vi "Send Message (Single).vi"(8 "error in (no error)":errorcluster, 9 "Delay Seconds":i32, 10 "Message Body":string, 11 "SQS in":refnum<class "Queue.lvclass">) -> (0 "error out":errorcluster, 1 "Message Body MD5":string, 2 "Message ID":string, 3 "SQS out":refnum<class "Queue.lvclass">)   [LabVIEW 2015, in "NI_AWS_SQS.lvlib" / "Queue.lvclass"]
uses:
  Queue.lvclass
  Core/HTTP Request/Name Value Pair.ctl
  Core/HTTP Request/Request Options.ctl
  Queue.lvclass/Queue.ctl
  Read Account Number.vi
  Read Name.vi
  Core/HTTP Request/HTTP Request.lvclass
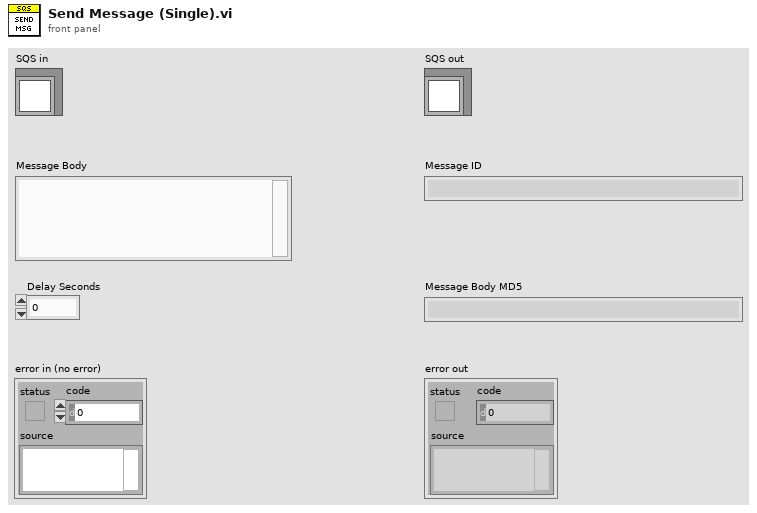
[diagram p1: front panel]
types:
  T1 = typedef "NI_AWS_Core.lvlib/HTTP Request.lvclass/Name Value Pair.ctl" = cluster{"name":string, "value":string}
  T2 = typedef "NI_AWS_Core.lvlib/HTTP Request.lvclass/Request Options.ctl" = cluster{"request headers":T1[], "request parameters":T1[], "request body":string}
  T3 = typedef "NI_AWS_Core.lvlib/HTTP Request.lvclass/Response.ctl" = cluster{"Headers":string, "Body":string}
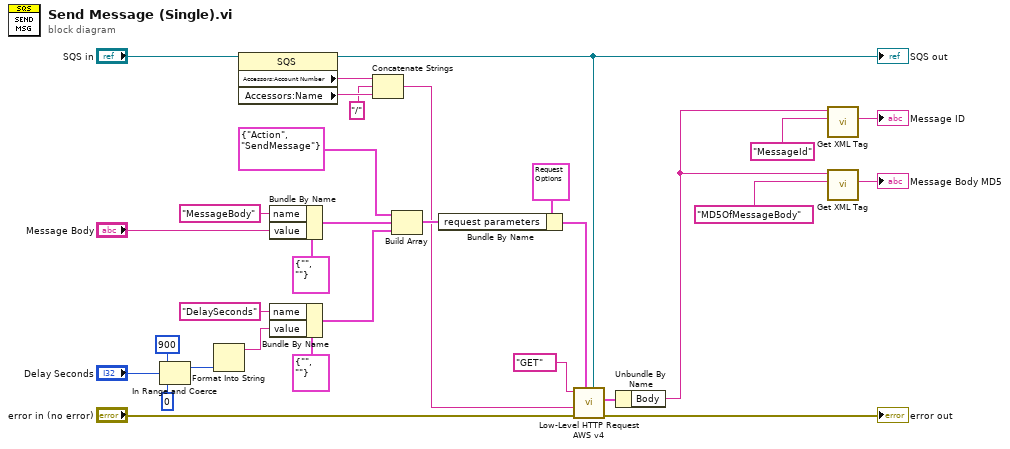
[diagram p0: block diagram]
diagram:
  n1 = In Range and Coerce(upper limit=900, x="Delay Seconds", lower limit=0) -> (coerced(x)=w3:i32)  [unwired: 1 out]
  n2 = Format Into String(w3) -> (resulting string=w5:string)  [unwired: 3 in, 1 out]
  n3 = property class="SQS"(reference="SQS in") -> (reference out=w22:refnum<class "Queue.lvclass">, "Accessors:Account Number"=w21:string, "Accessors:Name"=w20:string)  [unwired: 1 in, 1 out]
  "SQS out" <- w22
  n4 = Bundle By Name(cluster=T1 {"name"="", "value"=""} ("element"), "name"="MessageBody", "value"="Message Body") -> (w11:T1)
  n5 = Bundle By Name(cluster=T1 {"name"="", "value"=""} ("element"), "name"="DelaySeconds", "value"=w5) -> (w9:T1)
  n6 = Concatenate Strings(w21, "/", w20) -> (w18:string)
  n7 = Build Array(T1 {"name"="Action", "value"="SendMessage"} ("Cluster"), w11, w9) -> (w23:T1[])
  n8 = Bundle By Name(cluster=T2 {"request headers"=[], "request parameters"=[{"name"="Action", "value"="ListQueues"}], "request body"=""} ("Request Options"), "request parameters"=w23) -> (w24:T2)
  n9 = call "Low-Level HTTP Request AWS v4.vi"("AWS Core"=w22, "Request Options"=w24, "error in (no error)"="error in (no error)", "URL Suffix"=w18, "HTTP-Verb"="GET") -> ("error out"=→"error out":errorcluster, "Response"=w27:T3)  [unwired: 4 in, 1 out]
  n10 = Unbundle By Name(w27) -> ("Body"=w26:string)
  n11 = call "Get XML Tag.vi"("Tag name"="MessageId", "XML String in"=w26) -> ("Tag value"=→"Message ID":string)  [unwired: 5 in, 4 out]
  n12 = call "Get XML Tag.vi"("Tag name"="MD5OfMessageBody", "XML String in"=w26) -> ("Tag value"=→"Message Body MD5":string)  [unwired: 5 in, 4 out]
